vi "NOSO2 calc age.vi"(6 "PID":cluster{"P":dbl, "I":dbl, "Feed":dbl}, 8 "Flow Rate":dbl, 9 "NO/SO2 m ppm":dbl, 10 "NO/SO2 Conc":dbl, 11 "NO/SO2 t ppm":dbl) -> (2 "NO/SO2 MFR":dbl)   [LabVIEW 2014]
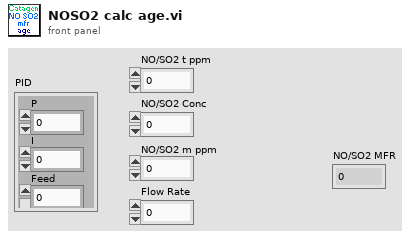
[diagram p1: front panel]
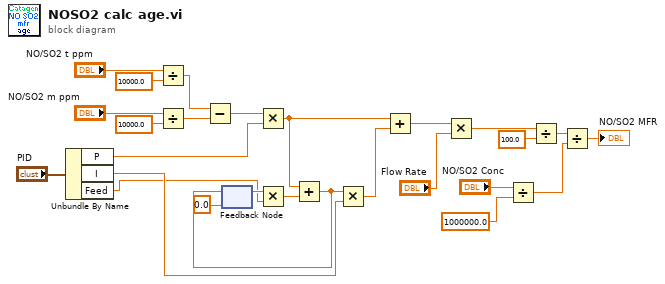
[diagram p0: block diagram]
diagram:
  n1 = Unbundle By Name("PID") -> ("P"=w3:dbl, "I"=w2:dbl, "Feed"=w1:dbl)
  n2 = Divide(x="NO/SO2 t ppm", y=10000.0) -> (x/y=w15:dbl)
  n3 = Divide(x="NO/SO2 m ppm", y=10000.0) -> (x/y=w16:dbl)
  n4 = Subtract(x=w15, y=w16) -> (x-y=w14:dbl)
  n5 = feedback #1(0.0) -> (w7:dbl)
  n6 = Multiply(x=w14, y=w3) -> (x*y=w12:dbl)
  n7 = Multiply(x=w7, y=w1) -> (x*y=w6:dbl)
  n8 = Add(x=w12, y=w6) -> (x+y=w8:dbl)
  n9 = feedback-in #1(w8) -> ()
  n10 = Multiply(x=w8, y=w2) -> (x*y=w11:dbl)
  n11 = Add(x=w12, y=w11) -> (x+y=w10:dbl)
  n12 = Multiply(x=w10, y="Flow Rate") -> (x*y=w21:dbl)
  n13 = Divide(x="NO/SO2 Conc", y=1000000.0) -> (x/y=w17:dbl)
  n14 = Divide(x=w21, y=100.0) -> (x/y=w20:dbl)
  n15 = Divide(x=w20, y=w17) -> (x/y=→"NO/SO2 MFR":dbl)
